vi "Measaurement_Conv.vi"(8 "error in (no error)":errorcluster, 11 "Measurements":T7) -> (0 "error in (no error)":errorcluster, 3 "Measurement JSON Data":T6 {"Ref ROI Cluster"."Edge Options ROI Ref"."Edge Polarity" items=["All Edges", "Rising Edges", "Falling Edges"]; "Ref ROI Cluster"."Edge Options ROI Ref"."Minimum Edge Strength" format="%.2f"; "Ref ROI Cluster"."Edge Options ROI Ref"."Width" step=2; "Ref ROI Cluster"."Edge Options ROI Ref"."Kernel Size" step=2; "Ref ROI Cluster"."Line Options ROI Ref"."Min. Points (%)" min=0.0 max=100.0; "Ref ROI Cluster"."Line Options ROI Ref"."Min. SNR (db)" min=0.0; "Ref ROI Cluster"."Line Options ROI Ref"."Max. Score" min=0.0 max=1024.0; "Ref ROI Cluster"."Line Options ROI Ref"."Min. Score" min=0.0 max=1024.0 step=1.0; "Measurement ROI 1 Cluster"."Meas ROI 1"."Contours"."Type" items=["No Selection", "Point", "Line", "Rectangle", "Oval", "Polygon", "Freehand Region", "Annulus", "Unused2", "Unused3", "Broken Line", "Freehand Line", "Rotated Rectangle"]; "Measurement ROI 1 Cluster"."Edge Options ROI 1"."Edge Polarity" items=["All Edges", "Rising Edges", "Falling Edges"]; "Measurement ROI 1 Cluster"."Edge Options ROI 1"."Minimum Edge Strength" format="%.2f"; "Measurement ROI 1 Cluster"."Edge Options ROI 1"."Width" step=2; "Measurement ROI 1 Cluster"."Edge Options ROI 1"."Kernel Size" step=2; "Measurement ROI 1 Cluster"."Line Options ROI 1"."Min. Points (%)" min=0.0 max=100.0; "Measurement ROI 1 Cluster"."Line Options ROI 1"."Min. SNR (db)" min=0.0; "Measurement ROI 1 Cluster"."Line Options ROI 1"."Max. Score" min=0.0 max=1024.0; "Measurement ROI 1 Cluster"."Line Options ROI 1"."Min. Score" min=0.0 max=1024.0 step=1.0; "Measurement ROI 1 Cluster"."Circle Options ROI 1"."Edge Options"."Edge Polarity" items=["All Edges", "Rising Edges", "Falling Edges"]; "Measurement ROI 1 Cluster"."Circle Options ROI 1"."Edge Options"."Minimum Edge Strength" format="%.2f"; "Measurement ROI 1 Cluster"."Circle Options ROI 1"."Edge Options"."Width" step=2; "Measurement ROI 1 Cluster"."Circle Options ROI 1"."Edge Options"."Kernel Size" step=2; "Measurement ROI 2 Cluster"."Meas ROI 2"."Contours"."Type" items=["No Selection", "Point", "Line", "Rectangle", "Oval", "Polygon", "Freehand Region", "Annulus", "Unused2", "Unused3", "Broken Line", "Freehand Line", "Rotated Rectangle"]; "Measurement ROI 2 Cluster"."Edge Options ROI 2"."Edge Polarity" items=["All Edges", "Rising Edges", "Falling Edges"]; "Measurement ROI 2 Cluster"."Edge Options ROI 2"."Minimum Edge Strength" format="%.2f"; "Measurement ROI 2 Cluster"."Edge Options ROI 2"."Width" step=2; "Measurement ROI 2 Cluster"."Edge Options ROI 2"."Kernel Size" step=2; "Measurement ROI 2 Cluster"."Line Options ROI 2"."Min. Points (%)" min=0.0 max=100.0; "Measurement ROI 2 Cluster"."Line Options ROI 2"."Min. SNR (db)" min=0.0; "Measurement ROI 2 Cluster"."Line Options ROI 2"."Max. Score" min=0.0 max=1024.0; "Measurement ROI 2 Cluster"."Line Options ROI 2"."Min. Score" min=0.0 max=1024.0 step=1.0; "Measurement ROI 2 Cluster"."Circle Options ROI 2"."Edge Options"."Edge Polarity" items=["All Edges", "Rising Edges", "Falling Edges"]; "Measurement ROI 2 Cluster"."Circle Options ROI 2"."Edge Options"."Minimum Edge Strength" format="%.2f"; "Measurement ROI 2 Cluster"."Circle Options ROI 2"."Edge Options"."Width" step=2; "Measurement ROI 2 Cluster"."Circle Options ROI 2"."Edge Options"."Kernel Size" step=2})   [LabVIEW 2019, in "Algorithm.lvclass"]
uses:
  FrameworkOverrides/Algorithm.lvclass
  <vilib>/vision/Measure.llb/Edge Polarity.ctl
  <vilib>/vision/Measure.llb/Edge Options.ctl
  <vilib>/vision/Measure.llb/Straight Edge Process.ctl
  <vilib>/vision/Measure.llb/Straight Edge Options.ctl
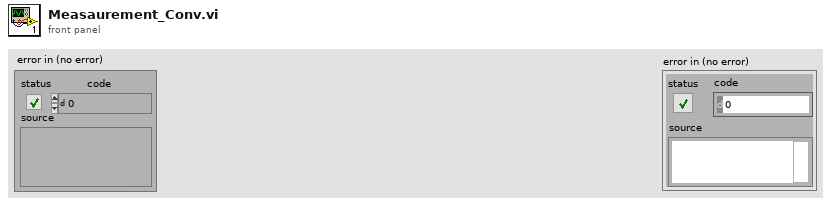
[diagram p1: front panel]
types:
  T1 = typedef "Edge Options.ctl" = cluster{"Edge Polarity":T2, "Kernel Size":u32, "Width":u32, "Minimum Edge Strength":sgl, "Interpolation Type":enum32{"Zero Order", "Bilinear", "Quadratic", "Cubic", "Bilinear Fixed"}, "Data Processing Method":enum32{"Average", "Median"}}
  T2 = typedef "Edge Polarity.ctl" = u32
  T3 = typedef "Straight Edge Options.ctl" = cluster{"Number of Lines":i32, "Type":T4, "Min. Score":dbl, "Max. Score":dbl, "Orientation":dbl, "Angle Range":dbl, "Angle Tolerance":dbl, "Step Size":u32, "Min. SNR (db)":dbl, "Min. Points (%)":dbl, "Hough Iterations":i32}
  T4 = typedef "Straight Edge Process.ctl" = enum32{"First Edge Rake", "Best Edge Rake", "Hough Edge Rake", "First Edge Projection", "Best Edge Projection"}
  T5 = typedef "ROI Descriptor" = cluster{"Global Rectangle":i32[], "Contours":cluster{"ID":enum32{"External", "Internal"}, "Type":u32, "Coordinates":i32[]}[]}
  T6 = cluster{"RackID":i32, "ImageID":i32, "CameraID":i32, "MeasurementID":i32, "Measurement Name":string, "Algo Name":string, "Algo Type":string, "Ref ROI Cluster":cluster{"ROI Ref":cluster{"Global Rectangle":i32[], "Contours":cluster{"ID":enum32{"External", "Internal"}, "Type":u32, "Coordinates":i32[]}[]}, "Edge Options ROI Ref":T1, "Line Options ROI Ref":T3, "Search Direction ROI Ref":u32, "RefROIEnable":bool}, "Measurement ROI 1 Cluster":cluster{"Meas ROI 1":T5, "Edge Options ROI 1":T1, "Line Options ROI 1":T3, "Scan/Search Direction ROI 1":u16, "Step Size ROI 1":u32, "Process ROI 1":enum16{"Get First Edge", "Get First + Last Edge", "Get All Edges", "Get Best Edge"}, "Circle Options ROI 1":cluster{"Search  Direction":u32, "Edge Options":T1, "Show Search Area":bool, "Show Search Lines":bool, "Show Edges Found":bool, "Show Result":bool, "Search Area Color":u32, "Search Lines Color":u32, "Edge Locations Color":u32, "Result Color":u32, "Overlay Group Name":string}, "Circle Fit Options ROI 1":cluster{"Process":enum16{"Get First Edge", "Get First + Last Edge", "Get All Edges", "Get Best Edge"}, "Step Size":dbl, "Max Pixel Radius":i32}}, "Measurement ROI 2 Cluster":cluster{"Meas ROI 2":T5, "Edge Options ROI 2":T1, "Line Options ROI 2":T3, "Scan/Search Direction ROI 2":u32, "Step Size ROI 2":u32, "Process ROI 2":enum16{"Get First Edge", "Get First + Last Edge", "Get All Edges", "Get Best Edge"}, "Circle Options ROI 2":cluster{"Search  Direction":u32, "Edge Options":T1, "Show Search Area":bool, "Show Search Lines":bool, "Show Edges Found":bool, "Show Result":bool, "Search Area Color":u32, "Search Lines Color":u32, "Edge Locations Color":u32, "Result Color":u32, "Overlay Group Name":string}, "Circle Fit Options ROI 2":cluster{"Process":enum16{"Get First Edge", "Get First + Last Edge", "Get All Edges", "Get Best Edge"}, "Step Size":dbl, "Max Pixel Radius":i32}}, "OverlayOptions":cluster{"OverlayEnable":bool, "OverlayText":string, "OverlayCoords":i32[], "OverlayAngle":i32, "OverlayTextSize":i32, "OverlayTextColor":string, "OverlayROI":bool, "OverlayRakeLine":bool, "OverlayPoints":bool}, "MathExpression":cluster{"Algorithm":string, "MathExpression":string, "ResultVariable":string}, "MathCorrectionParameters":cluster{"Radius":dbl, "CurlGap":dbl, "Thickness":dbl, "MeasurementIndices":i32[], "MathAlgoName":string, "MathAlgoFormula":string, "CorrectionForAngle":i32[], "NumericAray":i32[], "StringArray":string[]}, "ResultVariableCluster":cluster{"RVName":string, "RVSequence":string, "RVIndex":i32, "RVID":i32, "RVValue":dbl}, "CalibrationCoefficients":cluster{"A1":dbl, "A2":dbl, "A3":dbl}, cluster{"UserCalibCoefficients":cluster{"UserCorrectionLinearityCoeff":dbl, "UserCorrectionBiasCoeff":dbl}}, "SpecValues":cluster{"LCL":dbl, "UCL":dbl, "LSL":dbl, "USL":dbl, "NominalValue":dbl}}
  T7 = cluster{"RackID":i32, "ImageID":i32, "CameraID":i32, "MeasurementId":i32, "Name":string, "AlgoName":string, "Type":string, "MeasurementEnable":bool, "AlgorithmSequence":cluster{"RefernceEdge":cluster{"Enable":bool, "Method":string, "RefROI":cluster{"Left":i32, "Top":i32, "Right":i32, "Bottom":i32, "Rotation":dbl}, "EdgeOptions":cluster{"EdgePoarity":i32, "KernelSize":i32, "Width":i32, "MinimumEdgeStrength":i32, "InterpolationType":i32, "DataProcessingMethod":i32}, "LineOptions":cluster{"NumberofLines":i32, "Type":i32, "MinScore":i32, "MaxScore":i32, "Orientation":i32, "AngleRange":i32, "AngleTolerance":i32, "StepSize":i32, "MinSNR":i32, "MinPoints":i32, "HoughIterations":i32}, "SearchDirection":i32}, "Measurement":cluster{"ROI1":cluster{"Enable":bool, "ROI":cluster{"Left":i32, "Top":i32, "Right":i32, "Bottom":i32, "Rotation":dbl}, "EdgeOptions":cluster{"EdgePoarity":i32, "KernelSize":i32, "Width":i32, "MinimumEdgeStrength":i32, "InterpolationType":i32, "DataProcessingMethod":i32}, "LineOptions":cluster{"NumberofLines":i32, "Type":i32, "MinScore":i32, "MaxScore":i32, "Orientation":i32, "AngleRange":i32, "AngleTolerance":i32, "StepSize":i32, "MinSNR":i32, "MinPoints":i32, "HoughIterations":i32}, "Process":i32, "StepSize":i32, "SearchDirection":i32, "CircleEdgeOptions":cluster{"SearchDirection":i32, "EdgeOptions":cluster{"EdgePoarity":i32, "KernelSize":i32, "Width":i32, "MinimumEdgeStrength":i32, "InterpolationType":i32, "DataProcessingMethod":i32}}, "CircleFitOptions":cluster{"Process":i32, "StepSize":i32, "MAxPixelRadius":dbl}, "CircleSearchDirection":i32, "CurveParameters":cluster{"ExtractionMode":i32, "EdgeThreshold":i32, "EdgeFilterSize":i32, "MinLength":i32, "RowSearchStepSize":i32, "ColSearchStepSize":i32, "MaxEndpointGap":i32, "Closed":bool, "Subpixel":bool}, "MinimumMatchScore":i32, "CircleDescriptor":cluster{"MinRadius":i32, "MaxRadius":i32}, "EllipseDescriptor":cluster{"MinMajorRadius":i32, "MaxMajorRadius":i32, "MinMinorRadius":i32, "MaxMinorRadius":i32}}, "ROI2":cluster{"Enable":bool, "ROI":cluster{"Left":i32, "Top":i32, "Right":i32, "Bottom":i32, "Rotation":dbl}, "EdgeOptions":cluster{"EdgePoarity":i32, "KernelSize":i32, "Width":i32, "MinimumEdgeStrength":i32, "InterpolationType":i32, "DataProcessingMethod":i32}, "LineOptions":cluster{"NumberofLines":i32, "Type":i32, "MinScore":i32, "MaxScore":i32, "Orientation":i32, "AngleRange":i32, "AngleTolerance":i32, "StepSize":i32, "MinSNR":i32, "MinPoints":i32, "HoughIterations":i32}, "Process":i32, "StepSize":i32, "SearchDirection":i32, "CircleEdgeOptions":cluster{"SearchDirection":i32, "EdgeOptions":cluster{"EdgePoarity":i32, "KernelSize":i32, "Width":i32, "MinimumEdgeStrength":i32, "InterpolationType":i32, "DataProcessingMethod":i32}}, "CircleFitOptions":cluster{"Process":i32, "StepSize":i32, "MAxPixelRadius":dbl}, "CircleSearchDirection":i32, "CurveParameters":cluster{"ExtractionMode":i32, "EdgeThreshold":i32, "EdgeFilterSize":i32, "MinLength":i32, "RowSearchStepSize":i32, "ColSearchStepSize":i32, "MaxEndpointGap":i32, "Closed":bool, "Subpixel":bool}, "MinimumMatchScore":i32, "CircleDescriptor":cluster{"MinRadius":i32, "MaxRadius":i32}, "EllipseDescriptor":cluster{"MinMajorRadius":i32, "MaxMajorRadius":i32, "MinMinorRadius":i32, "MaxMinorRadius":i32}}}}, "MathExpression":cluster{"Algorithm":string, "MathExpression":string, "ResultVariable":string}, "MathCorrectionParameters":cluster{"Radius":dbl, "CurlGap":dbl, "Thickness":dbl, "MeasurementIndices":i32[], "MathAlgoName":string, "MathAlgoFormula":string, "CorrectionForAngle":i32[], "NumericAray":i32[], "StringArray":string[]}, "ResultVariableCluster":cluster{"RVName":string, "RVSequence":string, "RVIndex":i32, "RVID":i32, "RVValue":dbl}, "CalibrationCoefficients":cluster{"A1":dbl, "A2":dbl, "A3":dbl}, "UserCalibCoefficients":cluster{"UserCorrectionLinearityCoeff":dbl, "UserCorrectionBiasCoeff":dbl}, "SpecValues":cluster{"LCL":dbl, "UCL":dbl, "LSL":dbl, "USL":dbl, "NominalValue":dbl}, "OverlayOptions":cluster{"OverlayEnable":bool, "OverlayText":string, "OverlayCoords":i32[], "OverlayAngle":i32, "OverlayTextSize":i32, "OverlayTextColor":string, "OverlayROI":bool, "OverlayRakeLine":bool, "OverlayPoints":bool}, "DatalogEnable":bool, "DisplayIcon":string}
  T8 = cluster{"Search  Direction":u32, "Edge Options":T1, "Show Search Area":bool, "Show Search Lines":bool, "Show Edges Found":bool, "Show Result":bool, "Search Area Color":u32, "Search Lines Color":u32, "Edge Locations Color":u32, "Result Color":u32, "Overlay Group Name":string}
  T9 = cluster{"ROI Ref":cluster{"Global Rectangle":i32[], "Contours":cluster{"ID":enum32{"External", "Internal"}, "Type":u32, "Coordinates":i32[]}[]}, "Edge Options ROI Ref":T1, "Line Options ROI Ref":T3, "Search Direction ROI Ref":u32, "RefROIEnable":bool}
  T10 = cluster{"Meas ROI 2":T5, "Edge Options ROI 2":T1, "Line Options ROI 2":T3, "Scan/Search Direction ROI 2":u32, "Step Size ROI 2":u32, "Process ROI 2":enum16{"Get First Edge", "Get First + Last Edge", "Get All Edges", "Get Best Edge"}, "Circle Options ROI 2":cluster{"Search  Direction":u32, "Edge Options":T1, "Show Search Area":bool, "Show Search Lines":bool, "Show Edges Found":bool, "Show Result":bool, "Search Area Color":u32, "Search Lines Color":u32, "Edge Locations Color":u32, "Result Color":u32, "Overlay Group Name":string}, "Circle Fit Options ROI 2":cluster{"Process":enum16{"Get First Edge", "Get First + Last Edge", "Get All Edges", "Get Best Edge"}, "Step Size":dbl, "Max Pixel Radius":i32}}
  T11 = cluster{"Meas ROI 1":T5, "Edge Options ROI 1":T1, "Line Options ROI 1":T3, "Scan/Search Direction ROI 1":u16, "Step Size ROI 1":u32, "Process ROI 1":enum16{"Get First Edge", "Get First + Last Edge", "Get All Edges", "Get Best Edge"}, "Circle Options ROI 1":cluster{"Search  Direction":u32, "Edge Options":T1, "Show Search Area":bool, "Show Search Lines":bool, "Show Edges Found":bool, "Show Result":bool, "Search Area Color":u32, "Search Lines Color":u32, "Edge Locations Color":u32, "Result Color":u32, "Overlay Group Name":string}, "Circle Fit Options ROI 1":cluster{"Process":enum16{"Get First Edge", "Get First + Last Edge", "Get All Edges", "Get Best Edge"}, "Step Size":dbl, "Max Pixel Radius":i32}}
  T12 = cluster{"RefernceEdge":cluster{"Enable":bool, "Method":string, "RefROI":cluster{"Left":i32, "Top":i32, "Right":i32, "Bottom":i32, "Rotation":dbl}, "EdgeOptions":cluster{"EdgePoarity":i32, "KernelSize":i32, "Width":i32, "MinimumEdgeStrength":i32, "InterpolationType":i32, "DataProcessingMethod":i32}, "LineOptions":cluster{"NumberofLines":i32, "Type":i32, "MinScore":i32, "MaxScore":i32, "Orientation":i32, "AngleRange":i32, "AngleTolerance":i32, "StepSize":i32, "MinSNR":i32, "MinPoints":i32, "HoughIterations":i32}, "SearchDirection":i32}, "Measurement":cluster{"ROI1":cluster{"Enable":bool, "ROI":cluster{"Left":i32, "Top":i32, "Right":i32, "Bottom":i32, "Rotation":dbl}, "EdgeOptions":cluster{"EdgePoarity":i32, "KernelSize":i32, "Width":i32, "MinimumEdgeStrength":i32, "InterpolationType":i32, "DataProcessingMethod":i32}, "LineOptions":cluster{"NumberofLines":i32, "Type":i32, "MinScore":i32, "MaxScore":i32, "Orientation":i32, "AngleRange":i32, "AngleTolerance":i32, "StepSize":i32, "MinSNR":i32, "MinPoints":i32, "HoughIterations":i32}, "Process":i32, "StepSize":i32, "SearchDirection":i32, "CircleEdgeOptions":cluster{"SearchDirection":i32, "EdgeOptions":cluster{"EdgePoarity":i32, "KernelSize":i32, "Width":i32, "MinimumEdgeStrength":i32, "InterpolationType":i32, "DataProcessingMethod":i32}}, "CircleFitOptions":cluster{"Process":i32, "StepSize":i32, "MAxPixelRadius":dbl}, "CircleSearchDirection":i32, "CurveParameters":cluster{"ExtractionMode":i32, "EdgeThreshold":i32, "EdgeFilterSize":i32, "MinLength":i32, "RowSearchStepSize":i32, "ColSearchStepSize":i32, "MaxEndpointGap":i32, "Closed":bool, "Subpixel":bool}, "MinimumMatchScore":i32, "CircleDescriptor":cluster{"MinRadius":i32, "MaxRadius":i32}, "EllipseDescriptor":cluster{"MinMajorRadius":i32, "MaxMajorRadius":i32, "MinMinorRadius":i32, "MaxMinorRadius":i32}}, "ROI2":cluster{"Enable":bool, "ROI":cluster{"Left":i32, "Top":i32, "Right":i32, "Bottom":i32, "Rotation":dbl}, "EdgeOptions":cluster{"EdgePoarity":i32, "KernelSize":i32, "Width":i32, "MinimumEdgeStrength":i32, "InterpolationType":i32, "DataProcessingMethod":i32}, "LineOptions":cluster{"NumberofLines":i32, "Type":i32, "MinScore":i32, "MaxScore":i32, "Orientation":i32, "AngleRange":i32, "AngleTolerance":i32, "StepSize":i32, "MinSNR":i32, "MinPoints":i32, "HoughIterations":i32}, "Process":i32, "StepSize":i32, "SearchDirection":i32, "CircleEdgeOptions":cluster{"SearchDirection":i32, "EdgeOptions":cluster{"EdgePoarity":i32, "KernelSize":i32, "Width":i32, "MinimumEdgeStrength":i32, "InterpolationType":i32, "DataProcessingMethod":i32}}, "CircleFitOptions":cluster{"Process":i32, "StepSize":i32, "MAxPixelRadius":dbl}, "CircleSearchDirection":i32, "CurveParameters":cluster{"ExtractionMode":i32, "EdgeThreshold":i32, "EdgeFilterSize":i32, "MinLength":i32, "RowSearchStepSize":i32, "ColSearchStepSize":i32, "MaxEndpointGap":i32, "Closed":bool, "Subpixel":bool}, "MinimumMatchScore":i32, "CircleDescriptor":cluster{"MinRadius":i32, "MaxRadius":i32}, "EllipseDescriptor":cluster{"MinMajorRadius":i32, "MaxMajorRadius":i32, "MinMinorRadius":i32, "MaxMinorRadius":i32}}}}
  T13 = cluster{"OverlayEnable":bool, "OverlayText":string, "OverlayCoords":i32[], "OverlayAngle":i32, "OverlayTextSize":i32, "OverlayTextColor":string, "OverlayROI":bool, "OverlayRakeLine":bool, "OverlayPoints":bool}
  T14 = cluster{"Algorithm":string, "MathExpression":string, "ResultVariable":string}
  T15 = cluster{"Radius":dbl, "CurlGap":dbl, "Thickness":dbl, "MeasurementIndices":i32[], "MathAlgoName":string, "MathAlgoFormula":string, "CorrectionForAngle":i32[], "NumericAray":i32[], "StringArray":string[]}
  T16 = cluster{"RVName":string, "RVSequence":string, "RVIndex":i32, "RVID":i32, "RVValue":dbl}
  T17 = cluster{"LCL":dbl, "UCL":dbl, "LSL":dbl, "USL":dbl, "NominalValue":dbl}
  T18 = cluster{"Enable":bool, "Method":string, "RefROI":cluster{"Left":i32, "Top":i32, "Right":i32, "Bottom":i32, "Rotation":dbl}, "EdgeOptions":cluster{"EdgePoarity":i32, "KernelSize":i32, "Width":i32, "MinimumEdgeStrength":i32, "InterpolationType":i32, "DataProcessingMethod":i32}, "LineOptions":cluster{"NumberofLines":i32, "Type":i32, "MinScore":i32, "MaxScore":i32, "Orientation":i32, "AngleRange":i32, "AngleTolerance":i32, "StepSize":i32, "MinSNR":i32, "MinPoints":i32, "HoughIterations":i32}, "SearchDirection":i32}
  T19 = cluster{"ROI1":cluster{"Enable":bool, "ROI":cluster{"Left":i32, "Top":i32, "Right":i32, "Bottom":i32, "Rotation":dbl}, "EdgeOptions":cluster{"EdgePoarity":i32, "KernelSize":i32, "Width":i32, "MinimumEdgeStrength":i32, "InterpolationType":i32, "DataProcessingMethod":i32}, "LineOptions":cluster{"NumberofLines":i32, "Type":i32, "MinScore":i32, "MaxScore":i32, "Orientation":i32, "AngleRange":i32, "AngleTolerance":i32, "StepSize":i32, "MinSNR":i32, "MinPoints":i32, "HoughIterations":i32}, "Process":i32, "StepSize":i32, "SearchDirection":i32, "CircleEdgeOptions":cluster{"SearchDirection":i32, "EdgeOptions":cluster{"EdgePoarity":i32, "KernelSize":i32, "Width":i32, "MinimumEdgeStrength":i32, "InterpolationType":i32, "DataProcessingMethod":i32}}, "CircleFitOptions":cluster{"Process":i32, "StepSize":i32, "MAxPixelRadius":dbl}, "CircleSearchDirection":i32, "CurveParameters":cluster{"ExtractionMode":i32, "EdgeThreshold":i32, "EdgeFilterSize":i32, "MinLength":i32, "RowSearchStepSize":i32, "ColSearchStepSize":i32, "MaxEndpointGap":i32, "Closed":bool, "Subpixel":bool}, "MinimumMatchScore":i32, "CircleDescriptor":cluster{"MinRadius":i32, "MaxRadius":i32}, "EllipseDescriptor":cluster{"MinMajorRadius":i32, "MaxMajorRadius":i32, "MinMinorRadius":i32, "MaxMinorRadius":i32}}, "ROI2":cluster{"Enable":bool, "ROI":cluster{"Left":i32, "Top":i32, "Right":i32, "Bottom":i32, "Rotation":dbl}, "EdgeOptions":cluster{"EdgePoarity":i32, "KernelSize":i32, "Width":i32, "MinimumEdgeStrength":i32, "InterpolationType":i32, "DataProcessingMethod":i32}, "LineOptions":cluster{"NumberofLines":i32, "Type":i32, "MinScore":i32, "MaxScore":i32, "Orientation":i32, "AngleRange":i32, "AngleTolerance":i32, "StepSize":i32, "MinSNR":i32, "MinPoints":i32, "HoughIterations":i32}, "Process":i32, "StepSize":i32, "SearchDirection":i32, "CircleEdgeOptions":cluster{"SearchDirection":i32, "EdgeOptions":cluster{"EdgePoarity":i32, "KernelSize":i32, "Width":i32, "MinimumEdgeStrength":i32, "InterpolationType":i32, "DataProcessingMethod":i32}}, "CircleFitOptions":cluster{"Process":i32, "StepSize":i32, "MAxPixelRadius":dbl}, "CircleSearchDirection":i32, "CurveParameters":cluster{"ExtractionMode":i32, "EdgeThreshold":i32, "EdgeFilterSize":i32, "MinLength":i32, "RowSearchStepSize":i32, "ColSearchStepSize":i32, "MaxEndpointGap":i32, "Closed":bool, "Subpixel":bool}, "MinimumMatchScore":i32, "CircleDescriptor":cluster{"MinRadius":i32, "MaxRadius":i32}, "EllipseDescriptor":cluster{"MinMajorRadius":i32, "MaxMajorRadius":i32, "MinMinorRadius":i32, "MaxMinorRadius":i32}}}
  T20 = cluster{"Left":i32, "Top":i32, "Right":i32, "Bottom":i32, "Rotation":dbl}
  T21 = cluster{"EdgePoarity":i32, "KernelSize":i32, "Width":i32, "MinimumEdgeStrength":i32, "InterpolationType":i32, "DataProcessingMethod":i32}
  T22 = cluster{"NumberofLines":i32, "Type":i32, "MinScore":i32, "MaxScore":i32, "Orientation":i32, "AngleRange":i32, "AngleTolerance":i32, "StepSize":i32, "MinSNR":i32, "MinPoints":i32, "HoughIterations":i32}
  T23 = cluster{"Enable":bool, "ROI":cluster{"Left":i32, "Top":i32, "Right":i32, "Bottom":i32, "Rotation":dbl}, "EdgeOptions":cluster{"EdgePoarity":i32, "KernelSize":i32, "Width":i32, "MinimumEdgeStrength":i32, "InterpolationType":i32, "DataProcessingMethod":i32}, "LineOptions":cluster{"NumberofLines":i32, "Type":i32, "MinScore":i32, "MaxScore":i32, "Orientation":i32, "AngleRange":i32, "AngleTolerance":i32, "StepSize":i32, "MinSNR":i32, "MinPoints":i32, "HoughIterations":i32}, "Process":i32, "StepSize":i32, "SearchDirection":i32, "CircleEdgeOptions":cluster{"SearchDirection":i32, "EdgeOptions":cluster{"EdgePoarity":i32, "KernelSize":i32, "Width":i32, "MinimumEdgeStrength":i32, "InterpolationType":i32, "DataProcessingMethod":i32}}, "CircleFitOptions":cluster{"Process":i32, "StepSize":i32, "MAxPixelRadius":dbl}, "CircleSearchDirection":i32, "CurveParameters":cluster{"ExtractionMode":i32, "EdgeThreshold":i32, "EdgeFilterSize":i32, "MinLength":i32, "RowSearchStepSize":i32, "ColSearchStepSize":i32, "MaxEndpointGap":i32, "Closed":bool, "Subpixel":bool}, "MinimumMatchScore":i32, "CircleDescriptor":cluster{"MinRadius":i32, "MaxRadius":i32}, "EllipseDescriptor":cluster{"MinMajorRadius":i32, "MaxMajorRadius":i32, "MinMinorRadius":i32, "MaxMinorRadius":i32}}
  T24 = cluster{"SearchDirection":i32, "EdgeOptions":cluster{"EdgePoarity":i32, "KernelSize":i32, "Width":i32, "MinimumEdgeStrength":i32, "InterpolationType":i32, "DataProcessingMethod":i32}}
  T25 = cluster{"Process":i32, "StepSize":i32, "MAxPixelRadius":dbl}
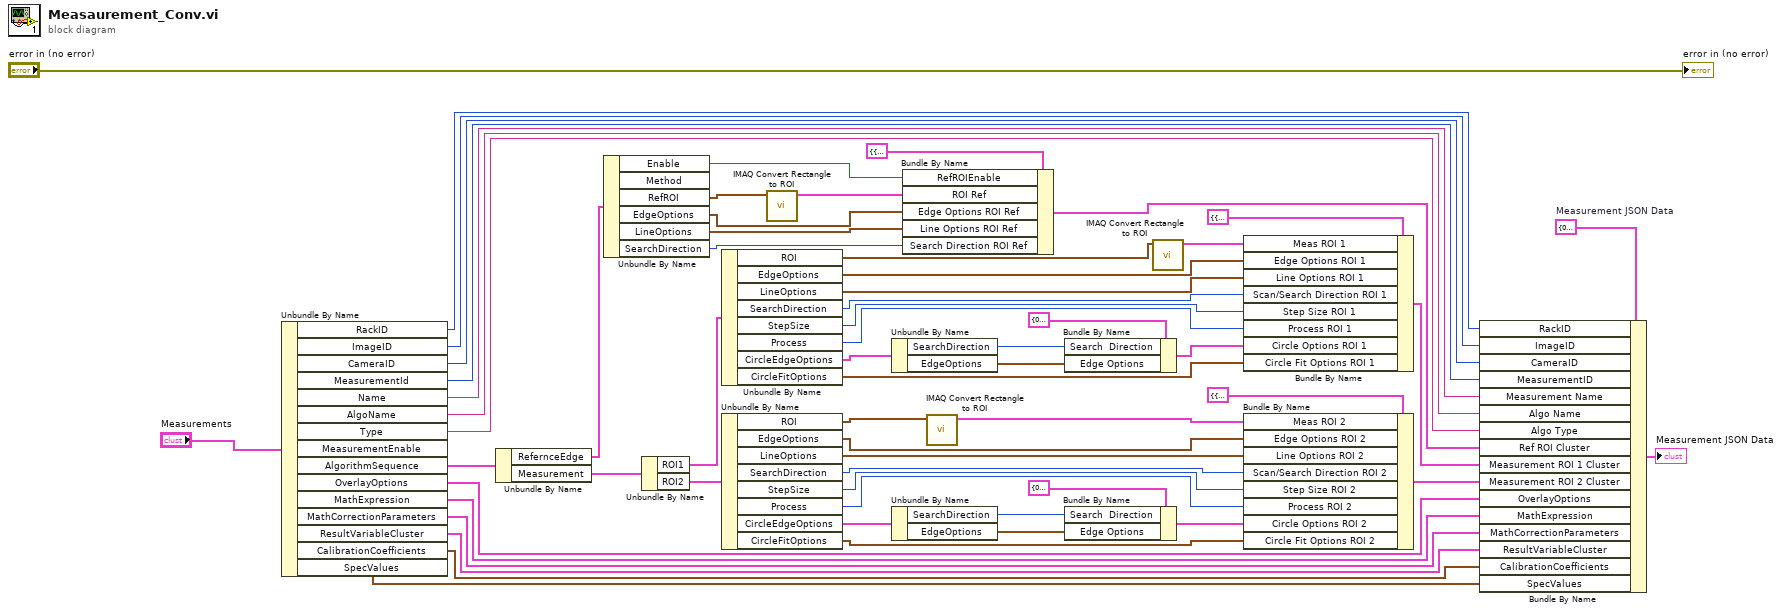
[diagram p0: block diagram]
diagram:
  w3 = T6 {"RackID"=0, "ImageID"=0, "CameraID"=0, "MeasurementID"=0, "Measurement Name"="", "Algo Name"="", "Algo Type"="", "Ref ROI Cluster"={"ROI Ref"={"Global Rectangle"=[], "Contours"=[]}, "Edge Options ROI Ref"={"Edge Polarity"=0, "Kernel Size"=3, "Width"=3, "Minimum Edge Strength"=10.0, "Interpolation Type"=enum."Bilinear Fixed", "Data Processing Method"=enum."Average"}, "Line Options ROI Ref"={"Number of Lines"=1, "Type"=enum."Best Edge Projection", "Min. Score"=0.0, "Max. Score"=1000.0, "Orientation"=0.0, "Angle Range"=5.0, "Angle Tolerance"=0.0, "Step Size"=5, "Min. SNR (db)"=0.0, "Min. Points (%)"=25.0, "Hough Iterations"=5}, "Search Direction ROI Ref"=0, "RefROIEnable"=FALSE}, "Measurement ROI 1 Cluster"={"Meas ROI 1"={"Global Rectangle"=[], "Contours"=[]}, "Edge Options ROI 1"={"Edge Polarity"=0, "Kernel Size"=3, "Width"=3, "Minimum Edge Strength"=10.0, "Interpolation Type"=enum."Bilinear Fixed", "Data Processing Method"=enum."Average"}, "Line Options ROI 1"={"Number of Lines"=1, "Type"=enum."Best Edge Projection", "Min. Score"=0.0, "Max. Score"=1000.0, "Orientation"=0.0, "Angle Range"=5.0, "Angle Tolerance"=0.0, "Step Size"=5, "Min. SNR (db)"=0.0, "Min. Points (%)"=25.0, "Hough Iterations"=5}, "Scan/Search Direction ROI 1"=0, "Step Size ROI 1"=0, "Process ROI 1"=enum."Get First Edge", "Circle Options ROI 1"={"Search  Direction"=0, "Edge Options"={"Edge Polarity"=0, "Kernel Size"=0, "Width"=0, "Minimum Edge Strength"=0.0, "Interpolation Type"=enum."Zero Order", "Data Processing Method"=enum."Average"}, "Show Search Area"=FALSE, "Show Search Lines"=FALSE, "Show Edges Found"=FALSE, "Show Result"=FALSE, "Search Area Color"=0, "Search Lines Color"=0, "Edge Locations Color"=0, "Result Color"=0, "Overlay Group Name"=""}, "Circle Fit Options ROI 1"={"Process"=enum."Get First Edge", "Step Size"=0.0, "Max Pixel Radius"=0}}, "Measurement ROI 2 Cluster"={"Meas ROI 2"={"Global Rectangle"=[], "Contours"=[]}, "Edge Options ROI 2"={"Edge Polarity"=0, "Kernel Size"=3, "Width"=3, "Minimum Edge Strength"=10.0, "Interpolation Type"=enum."Bilinear Fixed", "Data Processing Method"=enum."Average"}, "Line Options ROI 2"={"Number of Lines"=1, "Type"=enum."Best Edge Projection", "Min. Score"=0.0, "Max. Score"=1000.0, "Orientation"=0.0, "Angle Range"=5.0, "Angle Tolerance"=0.0, "Step Size"=5, "Min. SNR (db)"=0.0, "Min. Points (%)"=25.0, "Hough Iterations"=5}, "Scan/Search Direction ROI 2"=0, "Step Size ROI 2"=0, "Process ROI 2"=enum."Get First Edge", "Circle Options ROI 2"={"Search  Direction"=0, "Edge Options"={"Edge Polarity"=0, "Kernel Size"=0, "Width"=0, "Minimum Edge Strength"=0.0, "Interpolation Type"=enum."Zero Order", "Data Processing Method"=enum."Average"}, "Show Search Area"=FALSE, "Show Search Lines"=FALSE, "Show Edges Found"=FALSE, "Show Result"=FALSE, "Search Area Color"=0, "Search Lines Color"=0, "Edge Locations Color"=0, "Result Color"=0, "Overlay Group Name"=""}, "Circle Fit Options ROI 2"={"Process"=enum."Get First Edge", "Step Size"=0.0, "Max Pixel Radius"=0}}, "OverlayOptions"={"OverlayEnable"=FALSE, "OverlayText"="", "OverlayCoords"=[], "OverlayAngle"=0, "OverlayTextSize"=0, "OverlayTextColor"="", "OverlayROI"=FALSE, "OverlayRakeLine"=FALSE, "OverlayPoints"=FALSE}, "MathExpression"={"Algorithm"="", "MathExpression"="", "ResultVariable"=""}, "MathCorrectionParameters"={"Radius"=0.0, "CurlGap"=0.0, "Thickness"=0.0, "MeasurementIndices"=[], "MathAlgoName"="", "MathAlgoFormula"="", "CorrectionForAngle"=[], "NumericAray"=[], "StringArray"=[]}, "ResultVariableCluster"={"RVName"="", "RVSequence"="", "RVIndex"=0, "RVID"=0, "RVValue"=0.0}, "CalibrationCoefficients"={"A1"=0.0, "A2"=0.0, "A3"=0.0}, {"UserCalibCoefficients"={"UserCorrectionLinearityCoeff"=0.0, "UserCorrectionBiasCoeff"=0.0}}, "SpecValues"={"LCL"=0.0, "UCL"=0.0, "LSL"=0.0, "USL"=0.0, "NominalValue"=0.0}}  # Measurement JSON Data
  n1 = Unbundle By Name("Measurements") -> ("RackID"=w53:i32, "ImageID"=w52:i32, "CameraID"=w51:i32, "MeasurementId"=w50:i32, "Name"=w58:string, "AlgoName"=w57:string, "Type"=w56:string, "AlgorithmSequence"=w59:T12, "OverlayOptions"=w45:T13, "MathExpression"=w49:T14, "MathCorrectionParameters"=w48:T15, "ResultVariableCluster"=w47:T16, "CalibrationCoefficients"=w46:cluster{"A1":dbl, "A2":dbl, "A3":dbl}, "SpecValues"=w2:T17)  [unwired: 1 out]
  n2 = Unbundle By Name(w59) -> ("RefernceEdge"=w42:T18, "Measurement"=w33:T19)
  n3 = Unbundle By Name(w42) -> ("Enable"=w35:bool, "RefROI"=w40:T20, "EdgeOptions"=w38:T21, "LineOptions"=w37:T22, "SearchDirection"=w36:i32)  [unwired: 1 out]
  n4 = Unbundle By Name(w33) -> ("ROI1"=w32:T23, "ROI2"=w21:T23)
  n5 = Unbundle By Name(w32) -> ("ROI"=w31:T20, "EdgeOptions"=w29:T21, "LineOptions"=w28:T22, "SearchDirection"=w10:i32, "StepSize"=w9:i32, "Process"=w8:i32, "CircleEdgeOptions"=w27:T24, "CircleFitOptions"=w22:T25)
  n6 = Unbundle By Name(w21) -> ("ROI"=w20:T20, "EdgeOptions"=w18:T21, "LineOptions"=w17:T22, "SearchDirection"=w7:i32, "StepSize"=w6:i32, "Process"=w5:i32, "CircleEdgeOptions"=w15:T24, "CircleFitOptions"=w11:T25)
  n7 = call "IMAQ Convert Rectangle to ROI"("Rectangle"=w40) -> ("ROI Descriptor"=w39:T5)  [unwired: 8 in, 1 out]
  n8 = Unbundle By Name(w27) -> ("SearchDirection"=w24:i32, "EdgeOptions"=w23:T21)
  n9 = Unbundle By Name(w15) -> ("SearchDirection"=w16:i32, "EdgeOptions"=w12:T21)
  n10 = Bundle By Name(cluster=T9 {"ROI Ref"={"Global Rectangle"=[], "Contours"=[]}, "Edge Options ROI Ref"={"Edge Polarity"=0, "Kernel Size"=0, "Width"=0, "Minimum Edge Strength"=0.0, "Interpolation Type"=enum."Zero Order", "Data Processing Method"=enum."Average"}, "Line Options ROI Ref"={"Number of Lines"=0, "Type"=enum."First Edge Rake", "Min. Score"=0.0, "Max. Score"=0.0, "Orientation"=0.0, "Angle Range"=0.0, "Angle Tolerance"=0.0, "Step Size"=0, "Min. SNR (db)"=0.0, "Min. Points (%)"=0.0, "Hough Iterations"=0}, "Search Direction ROI Ref"=0, "RefROIEnable"=FALSE} ("Ref ROI Cluster"), "RefROIEnable"=w35, "ROI Ref"=w39, "Edge Options ROI Ref"=w38, "Line Options ROI Ref"=w37, "Search Direction ROI Ref"=w36) -> (w34:T9)
  n11 = call "IMAQ Convert Rectangle to ROI"("Rectangle"=w20) -> ("ROI Descriptor"=w19:T5)  [unwired: 8 in, 1 out]
  n12 = Bundle By Name(cluster=T8 {"Search  Direction"=0, "Edge Options"={"Edge Polarity"=0, "Kernel Size"=0, "Width"=0, "Minimum Edge Strength"=0.0, "Interpolation Type"=enum."Zero Order", "Data Processing Method"=enum."Average"}, "Show Search Area"=FALSE, "Show Search Lines"=FALSE, "Show Edges Found"=FALSE, "Show Result"=FALSE, "Search Area Color"=0, "Search Lines Color"=0, "Edge Locations Color"=0, "Result Color"=0, "Overlay Group Name"=""} ("Circle Options ROI 1"), "Search  Direction"=w24, "Edge Options"=w23) -> (w25:T8)
  n13 = Bundle By Name(cluster=T8 {"Search  Direction"=0, "Edge Options"={"Edge Polarity"=0, "Kernel Size"=0, "Width"=0, "Minimum Edge Strength"=0.0, "Interpolation Type"=enum."Zero Order", "Data Processing Method"=enum."Average"}, "Show Search Area"=FALSE, "Show Search Lines"=FALSE, "Show Edges Found"=FALSE, "Show Result"=FALSE, "Search Area Color"=0, "Search Lines Color"=0, "Edge Locations Color"=0, "Result Color"=0, "Overlay Group Name"=""} ("Circle Options ROI 1"), "Search  Direction"=w16, "Edge Options"=w12) -> (w14:T8)
  n14 = call "IMAQ Convert Rectangle to ROI"("Rectangle"=w31) -> ("ROI Descriptor"=w30:T5)  [unwired: 8 in, 1 out]
  n15 = Bundle By Name(cluster=T11 {"Meas ROI 1"={"Global Rectangle"=[], "Contours"=[]}, "Edge Options ROI 1"={"Edge Polarity"=0, "Kernel Size"=0, "Width"=0, "Minimum Edge Strength"=0.0, "Interpolation Type"=enum."Zero Order", "Data Processing Method"=enum."Average"}, "Line Options ROI 1"={"Number of Lines"=0, "Type"=enum."First Edge Rake", "Min. Score"=0.0, "Max. Score"=0.0, "Orientation"=0.0, "Angle Range"=0.0, "Angle Tolerance"=0.0, "Step Size"=0, "Min. SNR (db)"=0.0, "Min. Points (%)"=0.0, "Hough Iterations"=0}, "Scan/Search Direction ROI 1"=0, "Step Size ROI 1"=0, "Process ROI 1"=enum."Get First Edge", "Circle Options ROI 1"={"Search  Direction"=0, "Edge Options"={"Edge Polarity"=0, "Kernel Size"=0, "Width"=0, "Minimum Edge Strength"=0.0, "Interpolation Type"=enum."Zero Order", "Data Processing Method"=enum."Average"}, "Show Search Area"=FALSE, "Show Search Lines"=FALSE, "Show Edges Found"=FALSE, "Show Result"=FALSE, "Search Area Color"=0, "Search Lines Color"=0, "Edge Locations Color"=0, "Result Color"=0, "Overlay Group Name"=""}, "Circle Fit Options ROI 1"={"Process"=enum."Get First Edge", "Step Size"=0.0, "Max Pixel Radius"=0}} ("Measurement ROI 1 Cluster"), "Meas ROI 1"=w30, "Edge Options ROI 1"=w29, "Line Options ROI 1"=w28, "Scan/Search Direction ROI 1"=w10, "Step Size ROI 1"=w9, "Process ROI 1"=w8, "Circle Options ROI 1"=w25, "Circle Fit Options ROI 1"=w22) -> (w44:T11)
  n16 = Bundle By Name(cluster=T10 {"Meas ROI 2"={"Global Rectangle"=[], "Contours"=[]}, "Edge Options ROI 2"={"Edge Polarity"=0, "Kernel Size"=0, "Width"=0, "Minimum Edge Strength"=0.0, "Interpolation Type"=enum."Zero Order", "Data Processing Method"=enum."Average"}, "Line Options ROI 2"={"Number of Lines"=0, "Type"=enum."First Edge Rake", "Min. Score"=0.0, "Max. Score"=0.0, "Orientation"=0.0, "Angle Range"=0.0, "Angle Tolerance"=0.0, "Step Size"=0, "Min. SNR (db)"=0.0, "Min. Points (%)"=0.0, "Hough Iterations"=0}, "Scan/Search Direction ROI 2"=0, "Step Size ROI 2"=0, "Process ROI 2"=enum."Get First Edge", "Circle Options ROI 2"={"Search  Direction"=0, "Edge Options"={"Edge Polarity"=0, "Kernel Size"=0, "Width"=0, "Minimum Edge Strength"=0.0, "Interpolation Type"=enum."Zero Order", "Data Processing Method"=enum."Average"}, "Show Search Area"=FALSE, "Show Search Lines"=FALSE, "Show Edges Found"=FALSE, "Show Result"=FALSE, "Search Area Color"=0, "Search Lines Color"=0, "Edge Locations Color"=0, "Result Color"=0, "Overlay Group Name"=""}, "Circle Fit Options ROI 2"={"Process"=enum."Get First Edge", "Step Size"=0.0, "Max Pixel Radius"=0}} ("Measurement ROI 2 Cluster"), "Meas ROI 2"=w19, "Edge Options ROI 2"=w18, "Line Options ROI 2"=w17, "Scan/Search Direction ROI 2"=w7, "Step Size ROI 2"=w6, "Process ROI 2"=w5, "Circle Options ROI 2"=w14, "Circle Fit Options ROI 2"=w11) -> (w43:T10)
  n17 = Bundle By Name(cluster=w3, "RackID"=w53, "ImageID"=w52, "CameraID"=w51, "MeasurementID"=w50, "Measurement Name"=w58, "Algo Name"=w57, "Algo Type"=w56, "Ref ROI Cluster"=w34, "Measurement ROI 1 Cluster"=w44, "Measurement ROI 2 Cluster"=w43, "OverlayOptions"=w45, "MathExpression"=w49, "MathCorrectionParameters"=w48, "ResultVariableCluster"=w47, "CalibrationCoefficients"=w46, "SpecValues"=w2) -> (→"Measurement JSON Data":T6)
  "error in (no error)" <- "error in (no error)"
